vi "LINX - SPI Loopback.vi"() -> ()   [LabVIEW 2020]
doc: "This example demonstrates how to configure the SPI master and do a data loopback test using a LINX device."
uses:
  vi.lib/MakerHub/LINX/Private/Type Defs/Peripherals/SPI/SPI Configuration.ctl
  vi.lib/MakerHub/LINX/Private/Type Defs/Peripherals/SPI/SPI Bit Order.ctl
  vi.lib/MakerHub/LINX/Private/Type Defs/Peripherals/SPI/SPI Mode.ctl
  vi.lib/MakerHub/LINX/Public/Peripherals/SPI/SPI CS Config.ctl
  vi.lib/MakerHub/LINX/Private/Type Defs/Peripherals/SPI/SPI CS Logic Level.ctl
  vi.lib/MakerHub/LINX/Private/Device/Type Defs/TCP Config.ctl
  vi.lib/MakerHub/LINX/Public/Peripherals/SPI/SPI Write Read 1 Frame.vi
  vi.lib/MakerHub/LINX/Public/Peripherals/SPI/SPI Write Read N Frames.vi
  vi.lib/MakerHub/LINX/Private/Local IO/LinxSpiWriteRead.vi
  vi.lib/MakerHub/LINX/Public/Utilities/Check Channel.vi
  vi.lib/MakerHub/LINX/Public/Utilities/Open TCP.vi
  vi.lib/MakerHub/LINX/Private/Utilties/Generate Error.vi
  vi.lib/MakerHub/LINX/LMH-LINX.lvlib
  vi.lib/MakerHub/LINX/Private/Device/Device.lvlib
panel:
  in  "TCP Configuration":T1
  out "Read Data":u8[](array[numeric])
  in  "CS Configuration":T2={"CS Channel"=10, "CS Logic Level"=enum."Active Low"}
  in  "Write Data":u8[](array[numeric])=[9, 27, 19, 87] format="%.0x"
  out "Actual Clock Frequency":u32
  in  "Stop Button":bool
  in  "SPI Configuration":T4={"Clock Frequency"=1000000, "Bit Order"=enum."LSb First", "SPI Mode"=enum."Mode 0"}
  # "SPI Loop Back Example\n\nThis example demonstrates how to configure the SPI master and write one frame of SPI data.\n\nInstructions\n0. Connect (short) the SPI MOSI and MOSI pins.\n1. Select the COM Port associated with the LINX Device.\n2. Select the SPI Configuration.\n3. Select the CS Configuration.\n4. Click the Run Arrow.\n5. Enter some data in the Write Data control.  Notice the output on the Read Data indicator."
  # "LINX Device Settings"
  # "SPI Master Settings"
  # "SPI Write / Read Configruation"
  # "SPI Master Settings\n1. Set the target SPI clock frequency.  \n   The possible frequencies varies by device and the actual frequency used is returned.\n2. The bit order determines the order that the individual bits in each byte are shifted out.\n3. SPI Mode determines the clock polarity and phase. (View context help on the SPI Configure VI for more information)"
  # "SPI Write / Read Configuration\n1. Select the CS (chip select) DO channel.  The channel is automatically set as an output.\n2. Select the logic level for the CS pin.\n3. CS is automatically toggled each when the SPI Write / Read VI executes."
  # "SPI Write / Read Frame\n1. A 'frame' is one SPI transaction.  It starts when CS goes active and ends when CS returns to the idle state.\n2. A frame can be an arbitrary number for bytes in lenght.\n3. When using the SPI Write / Read VI in 1 Frame mode all data bytes are sent in a single frame.  For example if the data array contains 4 bytes all 4 bytes are sent as a single frame.\n4. When using the SPI Write / Read in N Frames mode the data bytes are divided into multiple frames.  \n    For example if the data array contains 4 bytes and the frame size is set to 2 the SPI Write / Read VI will send 2 frames of 2 bytes each.\n    The number of data bytes must be evenly divisble by the frame size."
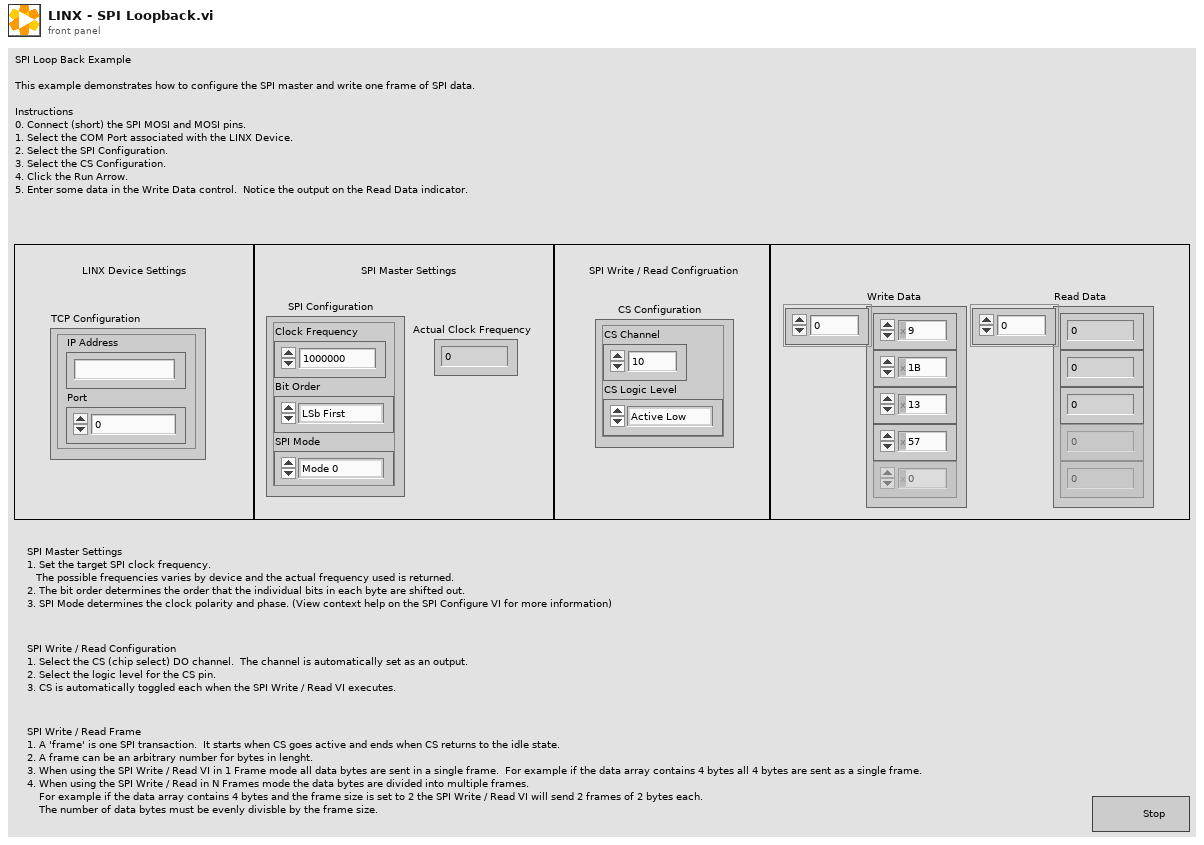
[diagram p1: front panel]
types:
  T1 = typedef "Device.lvlib/TCP Config.ctl" = cluster{"IP Address":string, "Port":u16}
  T2 = typedef "LMH-LINX.lvlib/SPI CS Config.ctl" = cluster{"CS Channel":u8, "CS Logic Level":T3}
  T3 = typedef "LMH-LINX.lvlib/SPI CS Logic Level.ctl" = enum8{"Active Low", "Active High"}
  T4 = typedef "LMH-LINX.lvlib/SPI Configuration.ctl" = cluster{"Clock Frequency":u32, "Bit Order":T5, "SPI Mode":T6}
  T5 = typedef "LMH-LINX.lvlib/SPI Bit Order.ctl" = enum8{"LSb First", "MSb First"}
  T6 = typedef "LMH-LINX.lvlib/SPI Mode.ctl" = enum8{"Mode 0", "Mode 1", "Mode 2", "Mode 3"}
  T7 = typedef "LMH-LINX.lvlib/LINX Ref.ctl" = cluster{"IO":T8, "Interface":T9, "LINX Device Config":T10}
  T8 = typedef "LMH-LINX.lvlib/Platform.ctl" = enum16{"Remote", "Local"}
  T9 = typedef "LMH-LINX.lvlib/Interface.ctl" = enum16{"Serial", "TCP"}
  T10 = typedef "Device.lvlib/LINX Device Config.ctl" = cluster{"Interface":T9, "COM Port":refnum<visa-resource-name>, "TCP Configuration":T1, "Device Family":u8, "Device ID":u8, "Device Name":string, "TCP Ref":refnum<k5>, "Channels":T11}
  T11 = typedef "LMH-LINX.lvlib/Channels.ctl" = cluster{"DI":u8[], "DO":u8[], "AI":u8[], "AO":u8[], "PWM":u8[], "QE":u8[], "UART":u8[], "I2C 2":u8[], "SPI":u8[], "CAN":u8[], "Servo":u8[], "AI Ref (V)":dbl, "AI Resolution (Bits)":u8, "AO Ref (V)":dbl, "AO Resolution (Bits)":u8}
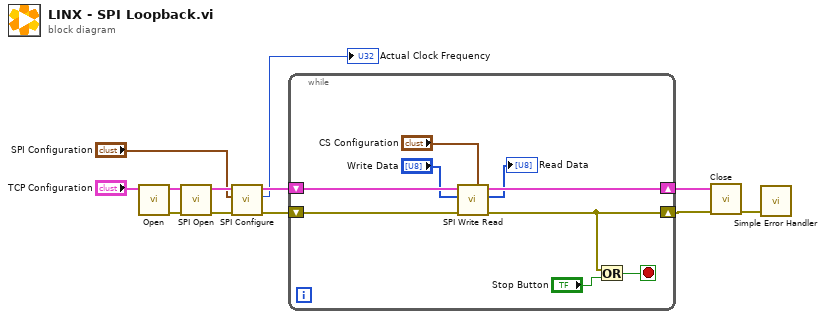
[diagram p0: block diagram]
diagram:
  n1 = call-poly "Open.vi"("TCP Configuration"="TCP Configuration") -> ("Error Out"=w9:errorcluster, "LINX Resource"=w12:T7)  [unwired: 8 in, 1 out]
  n2 = call "SPI Open.vi"("Error In"=w9, "LINX Resource"=w12) -> ("Error Out"=w10:errorcluster, "LINX Resource"=w11:T7)  [unwired: 8 in]
  n3 = call "SPI Configure.vi"("Error In"=w10, "SPI Configuration"="SPI Configuration", "LINX Resource"=w11) -> ("Error Out"=w6:errorcluster, "Actual Clock Frequency"=→"Actual Clock Frequency":u32, "LINX Resource"=w7:T7)  [unwired: 6 in]
  n4 = while {
    shift-right: [w16] -> w4
    shift-left: w6 -> [w20]
    shift-right: [w19] -> w5
    shift-left: w7 -> [w21]
    stop <- w18 stop-if-true
    n5 = call-poly "SPI Write Read.vi"("CS Configuration"="CS Configuration", "Error In"=w20, "Data"="Write Data", "LINX Resource"=w21) -> ("Error Out"=w16:errorcluster, "Read Data"=→"Read Data":u8[], "LINX Resource"=w19:T7)  [unwired: 4 in, 1 out]
    n6 = Or(x=w16, y="Stop Button") -> (x .or. y?=w18:bool)
  }
  n7 = call "Close.vi"("Error In"=w4, "LINX Resource"=w5) -> ("Error Out"=w2:errorcluster)  [unwired: 9 in]
  n8 = call <vilib>:"Simple Error Handler.vi"("error in (no error)"=w2) -> ()  [unwired: 4 in, 5 out]
